vi "S2DS_Error Pop-Up.vi"(8 "error constant":errorcluster, 10 "Send mail?":bool=TRUE) -> (0 "error constant (out)":errorcluster, 2 "Stop sweep?":bool)   [LabVIEW 2025]
uses:
  <vilib>/Utility/sysdir.llb/System Directory Type.ctl
  <vilib>/Utility/config.llb/Write Key (Boolean).vi
  <vilib>/Utility/config.llb/Write Key (String).vi
  <vilib>/Utility/config.llb/NI_LVConfig.lvlib
panel:
  in  "Clear error and stop sweep":bool
  in  "Clear error":bool
  out "Secondary message":string
  out "Main message":string
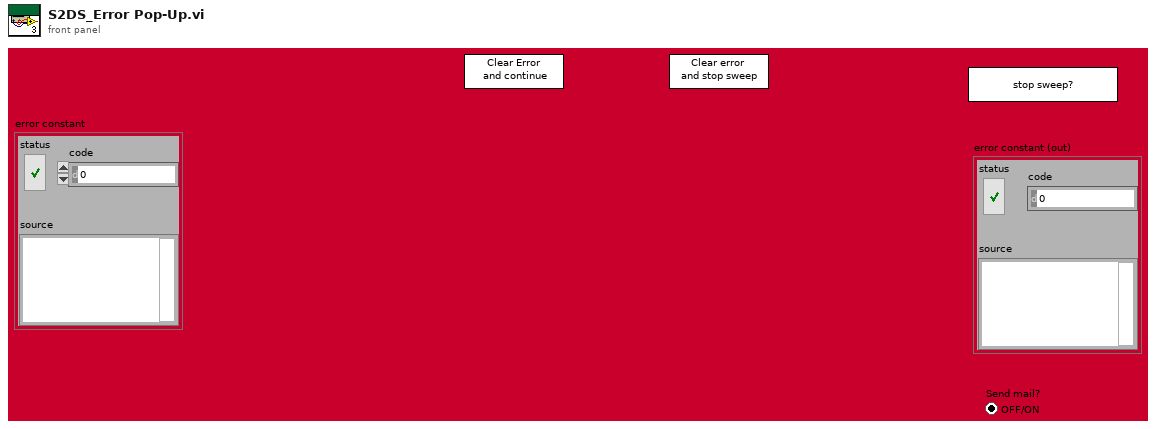
[diagram p1: front panel]
types:
  T1 = typedef "System Directory Type.ctl" = i32
  T2 = typedef "NI_LVConfig.lvlib/Config Data RefNum.ctl" = refnum<k1>
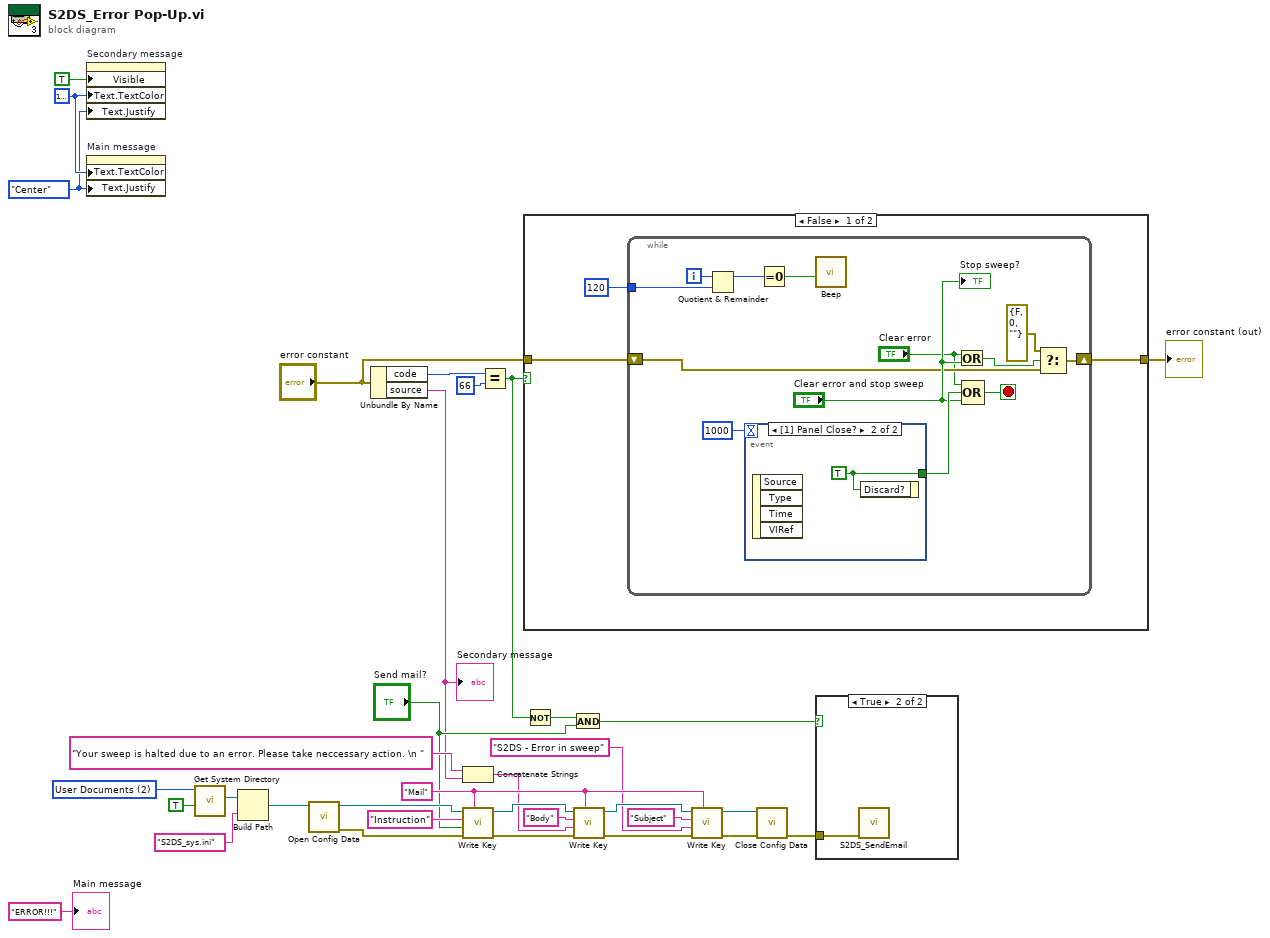
[diagram p0: block diagram]
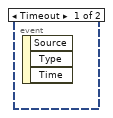
[diagram p2: hidden frame]
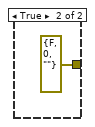
[diagram p3: hidden frame]
diagram:
  w14 = "Mail"
  w29 = T1 2 items=["User Home"=0, "User Desktop"=1, "User Documents"=2, "User Application Data"=3, "User Preferences"=4, "User Temporary"=5, "Public Documents"=6, "Public Application Data"=7, "Public Preferences"=8, "Public Cache"=13, "System Core Libraries"=9, "System Installed Libraries"=10, "Application Files"=11, "Boot Volume Root"=12] ("system directory type")
  w33 = u32 16777225 ("Text.Text Colors:Text Color")
  w32 = enum16{"Left", "Center", "Right"}."Center" ("Text.Justification")
  n1 = property on="Secondary message" class="Str"("Visible"=TRUE, "Text.TextColor"=w33, "Text.Justify"=w32) -> ()  [unwired: 2 in, 2 out]
  n2 = property on="Main message" class="Str"("Text.TextColor"=w33, "Text.Justify"=w32) -> ()  [unwired: 2 in, 2 out]
  n3 = call <vilib>:"Get System Directory.vi"("create directory if not found? (F)"=TRUE, "system directory type"=w29) -> ("system directory"=w27:path)  [unwired: 9 in]
  n4 = Build Path(base path=w27, name or relative path="S2DS_sys.ini") -> (appended path=w25:path)
  n5 = call <vilib>:"Open Config Data.vi"("configuration file path"=w25) -> ("error out"=w15:errorcluster, "refnum"=w24:T2)  [unwired: 8 in, 1 out]
  n6 = Unbundle By Name("error constant") -> ("code"=w9:i32, "source"=w1:string)
  "Secondary message" <- w1
  n7 = Concatenate Strings("Your sweep is halted due to an error. Please take neccessary action. \n ", w1) -> (w10:string)
  n8 = call-poly <vilib>:"Write Key.vi"("section"=w14, "error in (no error)"=w15, "value"="Send mail?", "key"="Instruction", "refnum"=w24) -> ("error out"=w17:errorcluster, "refnum out"=w23:T2)  [unwired: 4 in, 1 out]
  n9 = Equal?(x=w9, y=66) -> (x = y?=w2:bool)
  n10 = case shown="False" w2 {
    tunnel: [w37 errorcluster {"status"=FALSE, "code"=0, "source"=""} ("error constant")] -> w30
    tunnel: "error constant" -> [w36 _]
    frame False {
      n11 = while {
        tunnel: 120 -> [w47]
        shift-right: [w43] -> w37
        shift-left: w36 -> [w39]
        i -> [w50]
        stop <- w44 stop-if-true
        n12 = Quotient & Remainder(x=w50, y=w47) -> (x-y*floor(x/y)=w49:i32)  [unwired: 1 out]
        n13 = event shown="[1] Panel Close?" {
          selector: _ -> [_ _]
          dyn-events: _ -> [_ _]
          timeout: u32 1000 ("milliseconds to wait") -> [_ _]
          tunnel: [_ w51] -> w45
          event Timeout {
            n14 = event-data() -> ()  [unwired: 1 in, 3 out]
          }
          event Panel Close? {
            w51 = TRUE ("Discard?")
            n15 = event-data() -> ()  [unwired: 1 in, 4 out]
            n16 = event-data("Discard?"=w51) -> ()  [unwired: 1 in, 1 out]
          }
        }
        n17 = Equal To 0?(x=w49) -> (x = 0?=w48:bool)
        n18 = call <vilib>:"Beep.vi"("use system alert? (T)"=w48) -> ()  [unwired: 11 in]
        n19 = Or(x="Clear error", y="Clear error and stop sweep") -> (x .or. y?=w41:bool)
        n20 = Compound Arithmetic op=OR("Clear error", w45, "Clear error and stop sweep") -> (w44:bool)
        n21 = Select(t=errorcluster {"status"=FALSE, "code"=0, "source"=""}, s=w41, f=w39) -> (s? t:f=w43:errorcluster)
        "Stop sweep?" <- "Clear error and stop sweep"
      }
    }
    frame True {
    }
  }
  "error constant (out)" <- w30
  n22 = Not(x=w2) -> (.not. x?=w4:bool)
  n23 = And(x=w4, y="Send mail?") -> (x .and. y?=w3:bool)
  n24 = call-poly <vilib>:"Write Key.vi"("section"=w14, "error in (no error)"=w17, "value"=w10, "key"="Body", "refnum"=w23) -> ("error out"=w16:errorcluster, "refnum out"=w21:T2)  [unwired: 4 in, 1 out]
  n25 = call-poly <vilib>:"Write Key.vi"("section"=w14, "error in (no error)"=w16, "value"="S2DS - Error in sweep", "key"="Subject", "refnum"=w21) -> ("error out"=w18:errorcluster, "refnum out"=w19:T2)  [unwired: 4 in, 1 out]
  n26 = call <vilib>:"Close Config Data.vi"("error in (no error)"=w18, "refnum"=w19) -> ("error out"=w11:errorcluster)  [unwired: 8 in, 1 out]
  n27 = case shown="True" w3 {
    tunnel: w11 -> [_ w53]
    frame False {
    }
    frame True {
      n28 = call "S2DS_SendEmail.vi"("error in (no error)"=w53) -> ()  [unwired: 10 in, 1 out]
    }
  }
  "Main message" <- "ERROR!!!"
